vi "Configure Digital References .vi"(6 "Volts/Full Scale (1 Vrms)":dbl=1.0, 7 "Digital Audio Frequency (10 mHz)":dbl=10.0, 8 "error in (no error)":errorcluster, 9 "Decibel Reference B (1 dBrB)":dbl=1.0, 10 "Decibel Reference A (1 dBrA)":dbl=1.0, 11 "VISA resource name":refnum<visa-resource-name>) -> (0 "error out":errorcluster, 3 "VISA resource name out":refnum<visa-resource-name>)   [LabVIEW 2014, in "Stanford Research SR1.lvlib"]
doc: "Configures the Digital Reference settings."
uses:
  Stanford Research SR1.lvlib
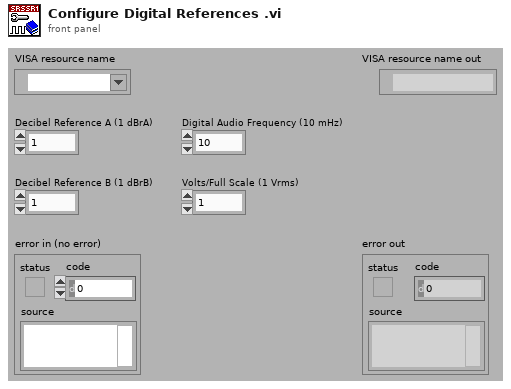
[diagram p1: front panel]
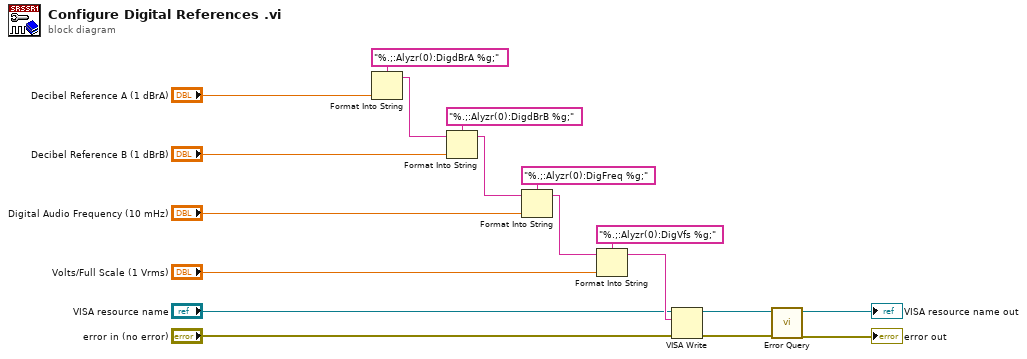
[diagram p0: block diagram]
diagram:
  n1 = Format Into String(format string="%.;:Alyzr(0):DigdBrA %g;", "Decibel Reference A (1 dBrA)") -> (resulting string=w16:string)  [unwired: 2 in, 1 out]
  n2 = Format Into String(format string="%.;:Alyzr(0):DigdBrB %g;", initial string=w16, "Decibel Reference B (1 dBrB)") -> (resulting string=w13:string)  [unwired: 1 in, 1 out]
  n3 = Format Into String(format string="%.;:Alyzr(0):DigFreq %g;", initial string=w13, "Digital Audio Frequency (10 mHz)") -> (resulting string=w10:string)  [unwired: 1 in, 1 out]
  n4 = Format Into String(format string="%.;:Alyzr(0):DigVfs %g;", initial string=w10, "Volts/Full Scale (1 Vrms)") -> (resulting string=w7:string)  [unwired: 1 in, 1 out]
  n5 = VISA Write(VISA resource name="VISA resource name", write buffer=w7, error in (no error)="error in (no error)") -> (VISA resource name out=w4:refnum<visa-resource-name>, error out=w3:errorcluster)  [unwired: 1 out]
  n6 = call "Error Query.vi"("error in (no error)"=w3, "VISA resource name"=w4) -> ("error out"=→"error out":errorcluster, "VISA resource name out"=→"VISA resource name out":refnum<visa-resource-name>)  [unwired: 6 in, 2 out]
